vi "Stop Reading.vi"() -> ()   [LabVIEW 2020]
panel:
  out "Stop Reading":bool
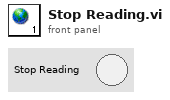
[diagram p1: front panel]
diagram:
